vi "Input Status Update.vi"(6 "Input Closed?":bool, 11 "Worker Block In":T1={"Block Status"=refnum, "Command Queue"=refnum, "Status"={"Block Status"={"State"=enum."Init", "Runs"=0, "i"=0, "Init"=FALSE, "Started"=FALSE, "Closing"=FALSE, "Phase"=enum."N/A", "Worker"=""}, "Error"={"status"=FALSE, "code"=0, "source"=""}}}) -> (1 "Block State":T4, 3 "Worker Block":T1={"Block Status"=refnum, "Command Queue"=refnum, "Status"={"Block Status"={"State"=enum."Init", "Runs"=0, "i"=0, "Init"=FALSE, "Started"=FALSE, "Closing"=FALSE, "Phase"=enum."N/A", "Worker"=""}, "Error"={"status"=FALSE, "code"=0, "source"=""}}})   [LabVIEW 2022 SP3, in "FlexBlocks Support.lvlib"]
uses:
  FlexBlocks Support.lvlib
  Block State.ctl
  Block Phase.ctl
  Block Status.ctl
  Block Command.ctl
  Block Status with Error.ctl
  Worker Block.ctl
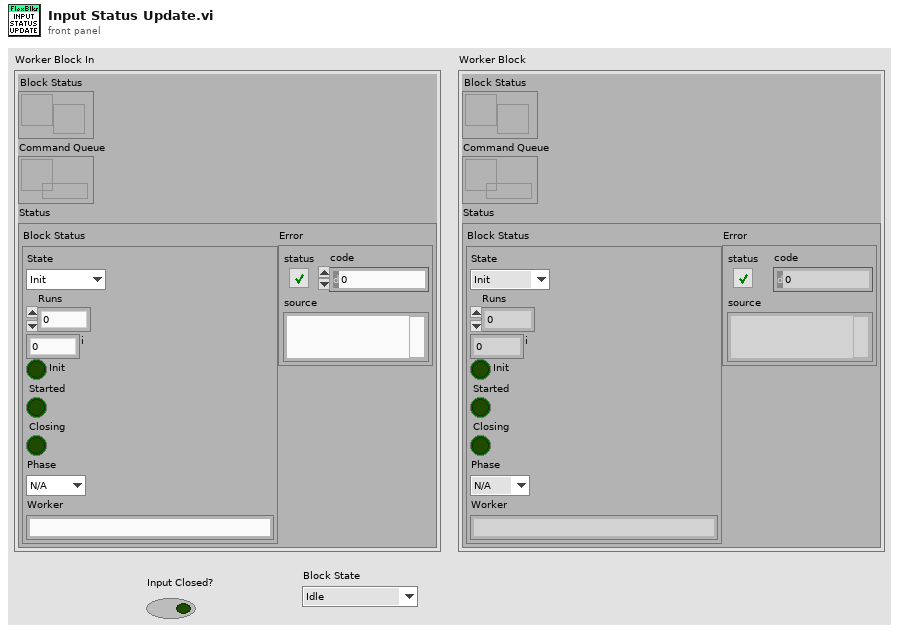
[diagram p1: front panel]
types:
  T1 = typedef "FlexBlocks Support.lvlib/Worker Block.ctl" = cluster{"Block Status":refnum<user-event>, "Command Queue":refnum<queue>, "Status":T2}
  T2 = typedef "FlexBlocks Support.lvlib/Block Status with Error.ctl" = cluster{"Block Status":T3, "Error":errorcluster}
  T3 = typedef "FlexBlocks Support.lvlib/Block Status.ctl" = cluster{"State":T4, "Runs":u32, "i":i32, "Init":bool, "Started":bool, "Closing":bool, "Phase":T5, "Worker":string}
  T4 = typedef "FlexBlocks Support.lvlib/Block State.ctl" = enum16{"Idle", "Init", "Start", "Run", "Stop", "Close"}
  T5 = typedef "FlexBlocks Support.lvlib/Block Phase.ctl" = enum16{"N/A", "Read", "Work", "Write"}
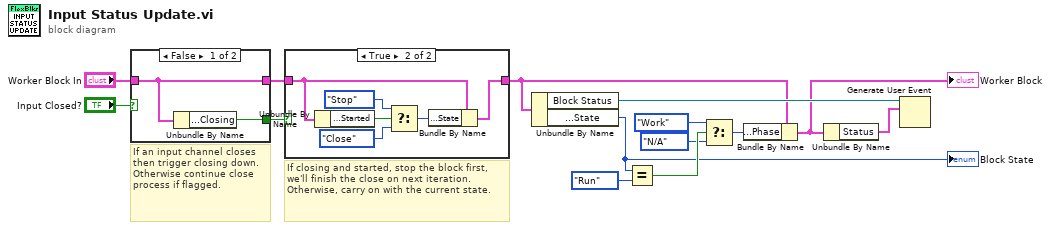
[diagram p0: block diagram]
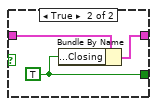
[diagram p3: hidden frame]
diagram:
  # "If closing and started, stop the block first, we'll finish the close on next iteration. Otherwise, carry on with the current state."
  # "If an input channel closes then trigger closing down. Otherwise continue close process if flagged."
  n1 = case shown="False" "Input Closed?" {
    tunnel: "Worker Block In" -> [w16 w19]
    tunnel: [w16 w18] -> w12
    tunnel: [w15 w17] -> w11
    frame False {
      n2 = Unbundle By Name(w16) -> ("Status.Block Status.Closing"=w15:bool)
    }
    frame True {
      w17 = TRUE ("Status.Block Status.Closing")
      n3 = Bundle By Name(cluster=w19, "Status.Block Status.Closing"=w17) -> (w18:T1)
    }
  }
  n4 = case shown="True" w11 {
    tunnel: w12 -> [w20 w23]
    tunnel: [w20 w21] -> w7
    frame False {
    }
    frame True {
      n5 = Unbundle By Name(w23) -> ("Status.Block Status.Started"=w25:bool)
      n6 = Select(t=Block_State."Stop" ("Block State"), s=w25, f=Block_State."Close" ("Block State")) -> (s? t:f=w22:T4)
      n7 = Bundle By Name(cluster=w23, "Status.Block Status.State"=w22) -> (w21:T1)
    }
  }
  n8 = Unbundle By Name(w7) -> ("Block Status"=w8:refnum<user-event>, "Status.Block Status.State"=w1:T4)
  "Block State" <- w1
  n9 = Equal?(x=w1, y=Block_State."Run") -> (x = y?=w9:bool)
  n10 = Select(t=Block_Phase."Work" ("Status.Block Status.Phase"), s=w9, f=Block_Phase."N/A" ("Status.Block Status.Phase")) -> (s? t:f=w4:T5)
  n11 = Bundle By Name(cluster=w7, "Status.Block Status.Phase"=w4) -> (w2:T1)
  "Worker Block" <- w2
  n12 = Unbundle By Name(w2) -> ("Status"=w3:T2)
  n13 = Generate User Event(user event=w8, event data cluster=w3) -> ()  [unwired: 2 in, 2 out]
